vi "Storage-wrapper.vi"(8 "error in":errorcluster, 10 "Storage element in":T1 {"Temperature characteristics"."Stand. dev. temperature" format="%#.1f"; "Temperature characteristics"."Min. temperature" format="%#.0f"; "Temperature characteristics"."Max. temperature" format="%#.0f"; "Temperature characteristics"."Average temperature" format="%#.0f"}, 11 "Storage params. ref. in":refnum<data-value>) -> (0 "error IO":errorcluster, 2 "Storage element":T1 {"Temperature characteristics"."Stand. dev. temperature" format="%#.1f"; "Temperature characteristics"."Min. temperature" format="%#.0f"; "Temperature characteristics"."Max. temperature" format="%#.0f"; "Temperature characteristics"."Average temperature" format="%#.0f"}, 3 "Storage params. ref.":refnum<data-value>)   [LabVIEW 2013, in "CameraVision.lvlib" / "CV-Main.lvclass"]
uses:
  CV-Main.lvclass
  Storage/CV-Storage.lvclass
  Buffers/Storage-buffer.ctl
  <vilib>/vision/Image Controls.llb/IMAQ Image.ctl
  Temperature/Temperature-characteristics.ctl
  Analysis/Characteristics-cluster.ctl
  Temperature/CV-Temperature.lvclass
  Analysis/CV-Analysis.lvclass
  Buffers/CV-Buffers.lvclass
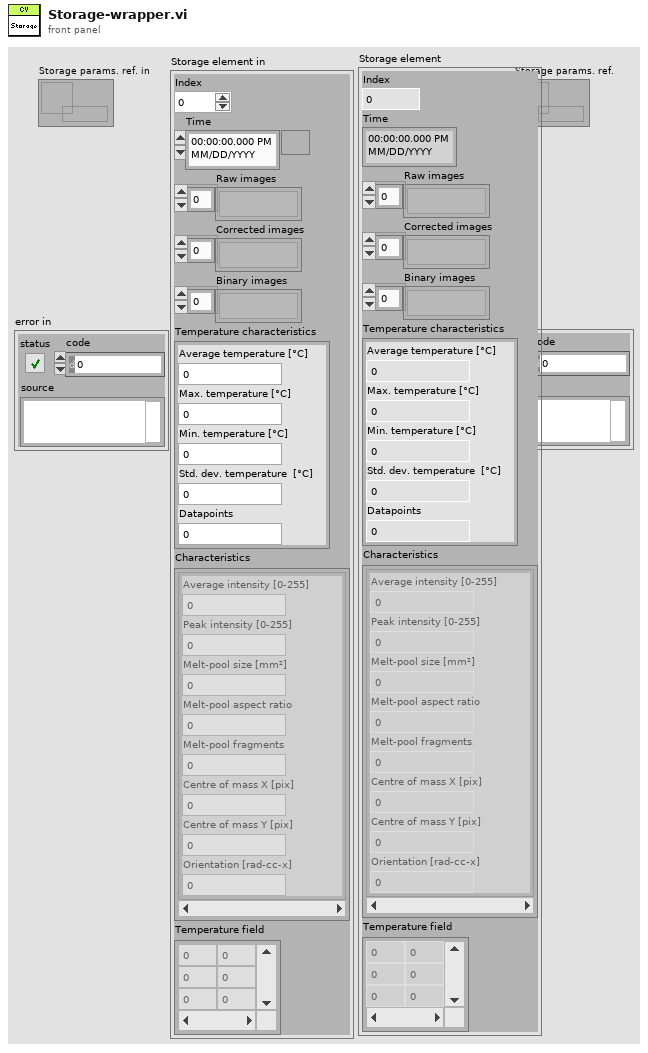
[diagram p1: front panel]
types:
  T1 = typedef "CameraVision.lvlib/CV-Buffers.lvclass/Storage-buffer.ctl" = cluster{"Index":i32, "Time":timestamp, "Raw images":T2[], "Corrected images":T2[], "Binary images":T2[], "Temperature characteristics":T3, "Characteristics":T4[], "Temperature field":dbl[][]}
  T2 = typedef "IMAQ Image.ctl" = refnum<image>
  T3 = typedef "CameraVision.lvlib/CV-Temperature.lvclass/Temperature-characteristics.ctl" = cluster{"Average temperature ":dbl, "Max. temperature":dbl, "Min. temperature":dbl, "Stand. dev. temperature":dbl, "Datapoints":dbl}
  T4 = typedef "CameraVision.lvlib/CV-Analysis.lvclass/Characteristics-cluster.ctl" = cluster{"Average intensity":dbl, "Peak intensity":dbl, "Melt-pool size":dbl, "Melt-pool aspect ratio":dbl, "Melt-pool fragments":dbl, "Centre of mass X":dbl, "Centre of mass Y":dbl, "Orientation":dbl}
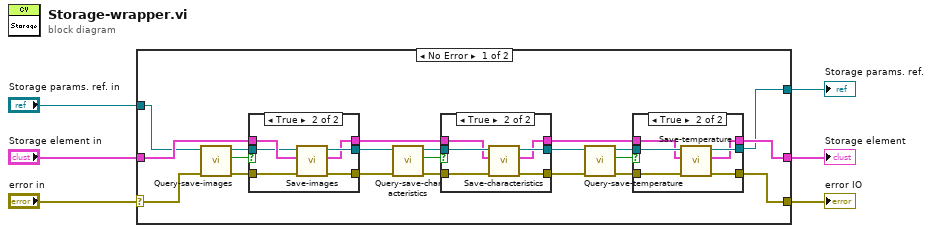
[diagram p0: block diagram]
diagram:
  n1 = case shown="No Error" "error in" {
    selector: "error in" -> [w8 w57]
    tunnel: [w13 w57] -> w5
    tunnel: "Storage params. ref. in" -> [w12 w56]
    tunnel: [w14 w56] -> w3
    tunnel: "Storage element in" -> [w16 w55]
    tunnel: [w15 w55] -> w1
    frame No Error {
      n2 = call "Query-save-images.vi"("error in"=w8, "Storage params. ref. in"=w12) -> ("error IO"=w9:errorcluster, "Save images?"=w10:bool, "Storage params. ref."=w11:refnum<data-value>)  [unwired: 7 in]
      n3 = case shown="True" w10 {
        tunnel: [w30 w36] -> w22
        tunnel: [w28 w35] -> w17
        tunnel: w16 -> [w29 w34]
        tunnel: w11 -> [w30 w33]
        tunnel: w9 -> [w28 w32]
        tunnel: [w29 w31] -> w7
        frame False {
        }
        frame True {
          n4 = call "Save-images.vi"("error in"=w32, "Storage element in"=w34, "Storage params. ref."=w33) -> ("error IO"=w35:errorcluster, "Storage element"=w31:T1, "Storage params. ref."=w36:refnum<data-value>)  [unwired: 6 in]
        }
      }
      n5 = call "Query-save-characteristics.vi"("error in"=w17, "Storage params. ref. in"=w22) -> ("error IO"=w25:errorcluster, "Save characteristics?"=w26:bool, "Storage params. ref."=w27:refnum<data-value>)  [unwired: 7 in]
      n6 = case shown="True" w26 {
        tunnel: w27 -> [w46 w54]
        tunnel: w25 -> [w48 w53]
        tunnel: [w48 w52] -> w19
        tunnel: w7 -> [w47 w51]
        tunnel: [w46 w50] -> w21
        tunnel: [w47 w49] -> w20
        frame False {
        }
        frame True {
          n7 = call "Save-characteristics.vi"("error in"=w53, "Storage element in"=w51, "Storage params. ref. in"=w54) -> ("error IO"=w52:errorcluster, "Storage element"=w49:T1, "Storage params. ref."=w50:refnum<data-value>)  [unwired: 6 in]
        }
      }
      n8 = call "Query-save-temperature.vi"("error in"=w19, "Storage params. ref. in"=w21) -> ("error IO"=w18:errorcluster, "Save temperature?"=w24:bool, "Storage params. ref."=w23:refnum<data-value>)  [unwired: 7 in]
      n9 = case shown="True" w24 {
        tunnel: w23 -> [w38 w45]
        tunnel: w18 -> [w39 w44]
        tunnel: [w39 w43] -> w13
        tunnel: w20 -> [w37 w42]
        tunnel: [w38 w41] -> w14
        tunnel: [w37 w40] -> w15
        frame False {
        }
        frame True {
          n10 = call "Save-temperature.vi"("error in"=w44, "Storage element in"=w42, "Storage params. ref. in"=w45) -> ("error IO"=w43:errorcluster, "Storage element"=w40:T1, "Storage params. ref."=w41:refnum<data-value>)  [unwired: 6 in]
        }
      }
    }
    frame Error {
    }
  }
  "error IO" <- w5
  "Storage params. ref." <- w3
  "Storage element" <- w1
